vi "Check if design exists.vi"(8 "error in":errorcluster, 11 "Request":T3={"Key"=["SERVER_PROTOCOL", "SERVER_SOFTWARE", "GATEWAY_INTERFACE", "SERVER_PORT", "SERVER_NAME", "DOCUMENT_ROOT", "SERVER_URL", "SERVER_ADDR", "SERVER_HOST", "QUERY_STRING", "CONTENT_LENGTH", "PATH_INFO", "SCRIPT_FILENAME", "AUTH_TYPE", "REMOTE_HOST", "SERVICE_NAME", "REQUEST_URI", "SERVICE_PATH", "REQUEST_TRANSPORT", "SCRIPT_NAME", "CONTENT_TYPE", "PATH_TRANSLATED", "REMOTE_USER", "REMOTE_ADDR", "REQUEST_METHOD", "CONTENT_LENGTH", "HOST", "CONNECTION", "REFERER", "ACCEPT", "COOKIE", "CACHE_CONTROL", "ACCEPT_ENCODING", "CONTENT_TYPE", "ACCEPT_CHARSET", "ACCEPT_LANGUAGE", "USER_AGENT", "ORIGIN", "HTTP_COOKIE", "ProjectCity", "FormName", "HL.Lfom[cm]", "Country", "ProjectTitle", "Email", "Name", "Organization", "Q.Plant[L/s]", "ProjectNotes", "ProjectState"], "Value"=["HTTP/1.1", "Mbedthis-Appweb/2.5.0", "CGI/1.1", "8080", "NI Application Web Server", "c:/program files/national instruments/shared/ni webserver/www", "NI Application Web Server", "", "NI Application Web Server", "", "216", "", "c:/program files/national instruments/shared/ni webserver/www/designserver/designform", "", "10.17.42.30", "designserver", "/DesignServer/DesignForm", "C:\\ProgramData\\National Instruments\\WebServices\\aws\\DesignServer-F226E305-64FF-4A12-B817-C09C85A5FBD8\\", "http", "/designserver/designform", "application/x-www-form-urlencoded", "", "", "10.17.42.30", "POST", "216", "designserver.cee.cornell.edu:8080", "keep-alive", "http://designserver.cee.cornell.edu/Designs/LFOM/Index.html", "text/html,application/xhtml+xml,application/xml;q=0.9,*/*;q=0.8", "__qca=P0-443584428-1305594823145; __unam=eda27ea-13048aaac3b-7928d9ad-1373; __utma=23486248.1568712313.1333468858.1342365063.1342378937.21; __utmz=23486248.1341744395.19.9.utmcsr=google|utmccn=(organic)|utmcmd=organic|utmctr=(not%20provided); __utma=67039164.2078665383.1313933611.1341311251.1342537309.26; __utmz=67039164.1341311251.25.3.utmcsr=courses.cornell.edu|utmccn=(referral)|utmcmd=referral|utmcct=/preview_program.php; cuwltgttime=\"1342815260\"; googtrans=/en/en; googtrans=/en/en", "max-age=0", "gzip,deflate,sdch", "application/x-www-form-urlencoded", "ISO-8859-1,utf-8;q=0.7,*;q=0.3", "en-US,en;q=0.8,es;q=0.6", "Mozilla/5.0 (Windows NT 6.1; WOW64) AppleWebKit/536.11 (KHTML, like Gecko) Chrome/20.0.1132.57 Safari/536.11", "http://designserver.cee.cornell.edu", "__qca=P0-443584428-1305594823145; __unam=eda27ea-13048aaac3b-7928d9ad-1373; __utma=23486248.1568712313.1333468858.1342365063.1342378937.21; __utmz=23486248.1341744395.19.9.utmcsr=google|utmccn=(organic)|utmcmd=organic|utmctr=(not%20provided); __utma=67039164.2078665383.1313933611.1341311251.1342537309.26; __utmz=67039164.1341311251.25.3.utmcsr=courses.cornell.edu|utmccn=(referral)|utmcmd=referral|utmcct=/preview_program.php; cuwltgttime=\"1342815260\"; googtrans=/en/en; googtrans=/en/en", "ITHACA", "LFOM", "20", "US", "", "mw24@cornell.edu", "Monroe Weber-Shirk", "Cornell University", "100", "", "New York"]}) -> (0 "error out":errorcluster, 1 "Method Version Folder":path, 2 "Design exists":bool, 3 "DesignRequest":T2, 5 "User and project info":T1)   [LabVIEW 2011]
uses:
  user project design.ctl
  Design Request.ctl
  Variable cluster.ctl
  Design Server.lvlib
panel:
  out "Design inputs 2":T1
  # "D:\\inetpub\\wwwroot\\Designs\\lfom\\5177\\342575026508"
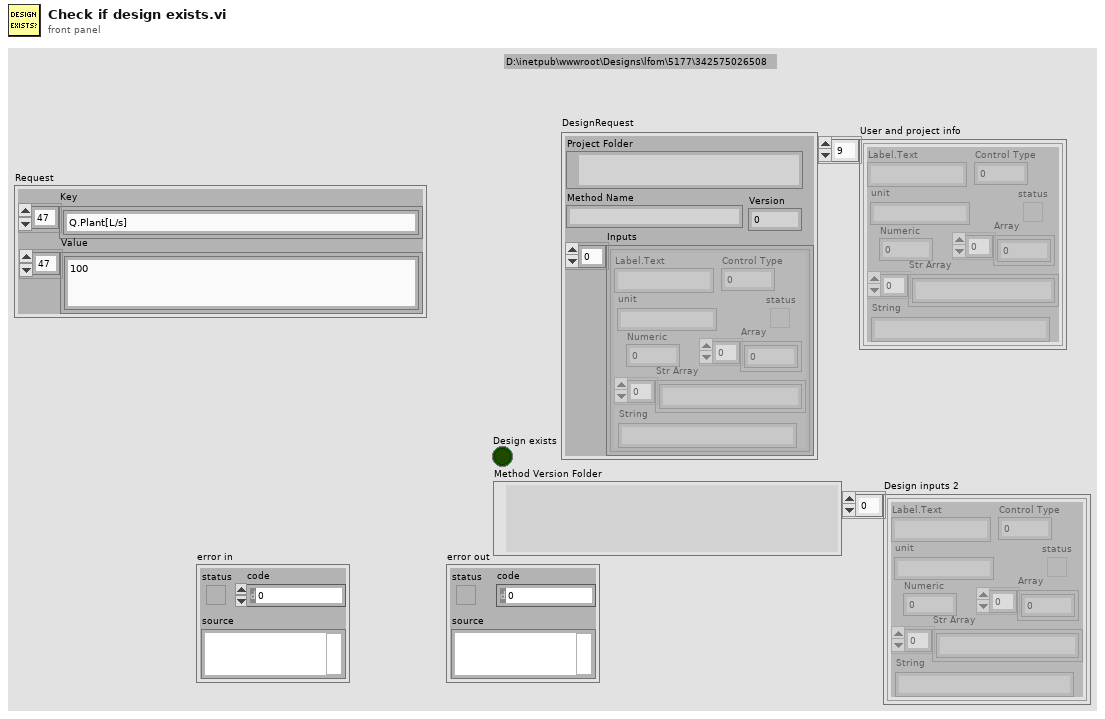
[diagram p1: front panel]
types:
  T1 = typedef "Design Server.lvlib/Variable cluster.ctl" = cluster{"Label.Text":string, "Control Type":u32, "Numeric":dbl, "Array":dbl[], "status":bool, "Str Array":string[], "String":string, "unit":string}[]
  T2 = typedef "Design Server.lvlib/Design Request.ctl" = cluster{"Project Folder":path, "Method Name":string, "Inputs":T1, "Version":i32}
  T3 = typedef "Design Server.lvlib/user project design.ctl" = cluster{"Key":string[], "Value":string[]}
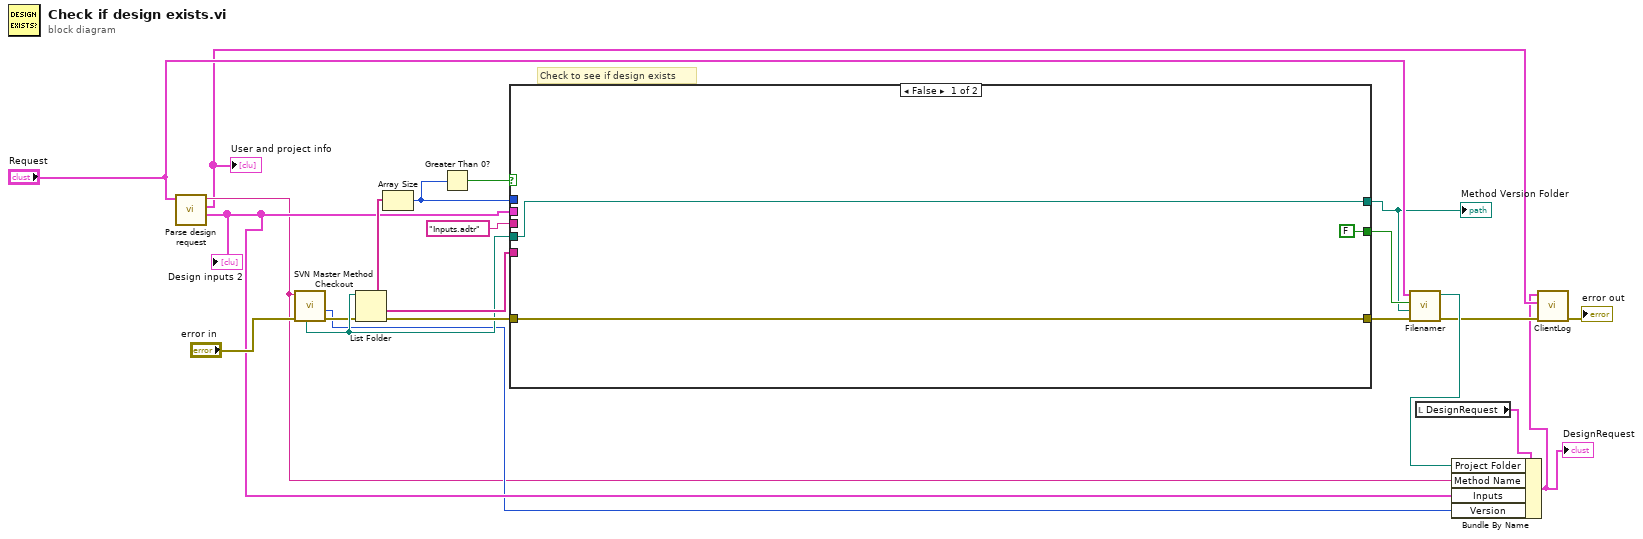
[diagram p0: block diagram]
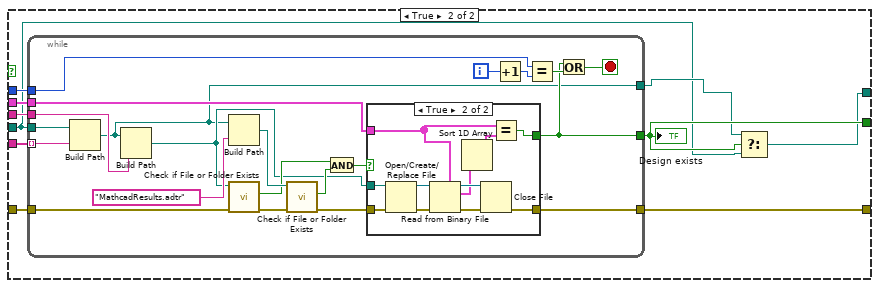
[diagram p2: hidden frame]
diagram:
  # "Check to see if design exists"
  n1 = call "Parse design request.vi"("Request"="Request") -> ("Design inputs"=w12:T1, "User and project info"=w2:T1, "Method"=w10:string)  [unwired: 7 in, 1 out]
  "Design inputs 2" <- w12
  "User and project info" <- w2
  n2 = call "SVN Master Method Checkout.vi"("error in (no error)"="error in", "Method Name"=w10) -> ("error out"=w14:errorcluster, "Method Version"=w11:i32, "method version folder"=w16:path)  [unwired: 4 in, 3 out]
  n3 = List Folder(path=w16, error in=w14) -> (folder names=w20:string[], error out=w21:errorcluster)  [unwired: 2 in, 2 out]
  n4 = Array Size(array=w20) -> (size(s)=w18:i32)
  n5 = Greater Than 0?(x=w18) -> (x > 0?=w19:bool)
  n6 = case shown="False" w19 {
    tunnel: w16 -> [w22 w25]
    tunnel: "Inputs.adtr" ("name or relative path") -> [_ w34]
    tunnel: w21 -> [w24 w33]
    tunnel: w20 -> [_ w32]
    tunnel: w18 -> [_ w31]
    tunnel: w12 -> [_ w30]
    tunnel: [w24 w29] -> w8
    tunnel: [FALSE w28] -> w9
    tunnel: [w22 w26] -> w6
    frame False {
    }
    frame True {
      n7 = while {
        tunnel: w25 -> [w55]
        tunnel: w32 -> [w54] mode=indexing
        tunnel: w34 -> [w53]
        tunnel: w33 -> [w46]
        tunnel: w31 -> [w44]
        tunnel: w30 -> [w40]
        tunnel: [w38] -> w28
        tunnel: [w36] -> w27
        tunnel: [w35] -> w29
        i -> [w45]
        stop <- w42 stop-if-true
        n8 = Build Path(base path=w55, name or relative path=w54) -> (appended path=w36:path)
        n9 = Build Path(base path=w36, name or relative path=w53) -> (appended path=w37:path)
        n10 = Build Path(base path=w36, name or relative path="MathcadResults.adtr") -> (appended path=w52:path)
        n11 = call <vilib>:"Check if File or Folder Exists.vi"("error in (no error)"=w46, "path"=w37) -> ("error out"=w47:errorcluster, "file or folder exists?"=w49:bool)  [unwired: 7 in, 1 out]
        n12 = call <vilib>:"Check if File or Folder Exists.vi"("error in (no error)"=w47, "path"=w52) -> ("error out"=w48:errorcluster, "file or folder exists?"=w50:bool)  [unwired: 7 in, 1 out]
        n13 = And(x=w49, y=w50) -> (x .and. y?=w39:bool)
        n14 = case shown="True" w39 {
          selector: w39 -> [w57 _]
          tunnel: w48 -> [w56 w66]
          tunnel: w40 -> [_ w63]
          tunnel: [w57 w62] -> w38
          tunnel: w37 -> [_ w61]
          tunnel: [w56 w60] -> w35
          frame False {
          }
          frame True {
            n15 = Open/Create/Replace File(file path (use dialog)=w61, error in=w66) -> (refnum out=w64:refnum<file>, error out=w68:errorcluster)  [unwired: 4 in, 1 out]
            n16 = Read from Binary File(5:w63, 8:w68, 11:w64) -> (0:w67:errorcluster, 2:w59:T1, 3:w65:refnum<file>)  [unwired: 3 in, 1 out]
            n17 = Sort 1D Array(array=w59) -> (sorted array=w58:T1)
            n18 = Close File(refnum=w65, error in=w67) -> (error out=w60:errorcluster)  [unwired: 1 out]
            n19 = Equal?(x=w63, y=w58) -> (x = y?=w62:bool)
          }
        }
        n20 = Increment(x=w45) -> (x+1=w41:i32)
        n21 = Equal?(x=w44, y=w41) -> (x = y?=w43:bool)
        n22 = Or(x=w38, y=w43) -> (x .or. y?=w42:bool)
      }
      "Design exists" <- w28
      n23 = Select(t=w27, s=w28, f=w25) -> (s? t:f=w26:path)
    }
  }
  "Method Version Folder" <- w6
  n24 = call "Filenamer.vi"("error in"=w8, "Method Version Folder"=w6, "Design exists"=w9, "request variables"="Request") -> ("error out"=w4:errorcluster, "Project Folder"=w5:path)  [unwired: 6 in]
  n25 = local read "DesignRequest"() -> (w13:T2)
  n26 = Bundle By Name(cluster=w13, "Project Folder"=w5, "Method Name"=w10, "Inputs"=w12, "Version"=w11) -> (w1:T2)
  "DesignRequest" <- w1
  n27 = call "ClientLog.vi"("error in (no error)"=w4, "User and Project Inputs"=w2, "DesignRequest"=w1) -> ("error out"=→"error out":errorcluster)  [unwired: 8 in]
